vi "MIF_auto_X_num-de-obs_discr.vi"(1 "xi-obs-num":dbl[](array[numeric])) -> (0 "xi-MIF-num":dbl[](array[numeric]))   [LabVIEW 2010, in "lv_02.lvlib"]
doc: "Pour une variable quantitative discrète (num-D), à partir du tableau xi-obs des n observations, le VI retourne un tableau xi-MIF des valeurs distinctes observées"
uses:
  lv_02.lvlib
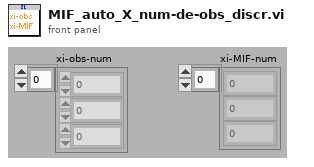
[diagram p1: front panel]
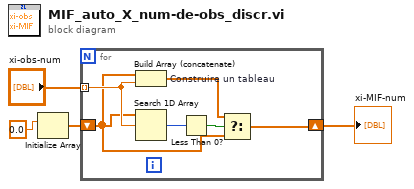
[diagram p0: block diagram]
diagram:
  n1 = Initialize Array(0.0) -> (w2:dbl[])  [unwired: 1 in]
  n2 = for {
    tunnel: "xi-obs-num" -> [w9] mode=indexing
    shift-right: [w6] -> w4
    shift-left: w2 -> [w7]
    n3 = Build Array (concatenate) "Construire un tableau"(w7, w9) -> (w8:dbl[])
    n4 = Search 1D Array(1D array=w7, element=w9) -> (index of element=w10:i32)  [unwired: 1 in]
    n5 = Less Than 0?(x=w10) -> (x < 0?=w5:bool)
    n6 = Select(t=w8, s=w5, f=w7) -> (s? t:f=w6:dbl[])
  }
  "xi-MIF-num" <- w4
